vi "蜂鸣器.vi"   [LabVIEW 2016]
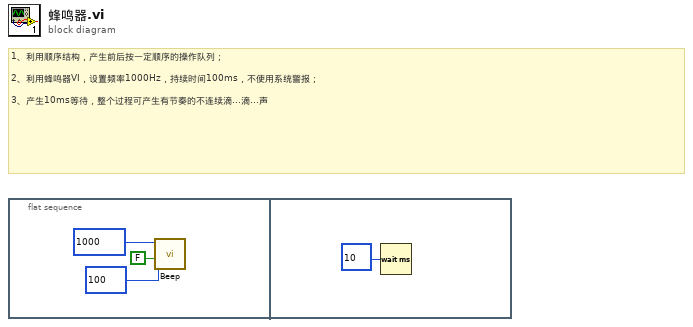
[diagram p0: block diagram]
diagram:
  # "1、利用顺序结构，产生前后按一定顺序的操作队列；\n\n2、利用蜂鸣器VI，设置频率1000Hz，持续时间100ms，不使用系统警报；\n\n3、产生10ms等待，整个过程可产生有节奏的不连续滴...滴...声"
  n1 = flat-sequence {
    frame #0 {
      n2 = call <vilib>:"Beep.vi"("use system alert? (T)"=FALSE, "duration (msec)"=u32 100, "frequency (Hz)"=u32 1000) -> ()  [unwired: 9 in]
    }
    frame #1 {
      n3 = Wait (ms)(milliseconds to wait=u32 10 ("等待时间（毫秒）")) -> ()  [unwired: 1 out]
    }
  }
